vi "SetTreeTags__slk_mt.vi"(8 "error in (no error)":errorcluster, 9 "parents symbol (-)":string="-", 10 "tags in":string[](array[string]), 11 "tree view in":refnum<class "TreeView__slk_mt.lvclass">) -> (0 "error out":errorcluster, 3 "tree view out":refnum<class "TreeView__slk_mt.lvclass">)   [LabVIEW 2020, in "TreeView__slk_mt.lvclass"]
doc: "Sets tags to a tree view objects."
uses:
  TreeView__slk_mt.lvclass
  TreeView__slk_mt.lvclass/TreeView__slk_mt.ctl
panel:
  # "SetTreeTags__slk_mt.vi\nSets tags to a tree view objects.\n\nNOTICE -- YOU MUST LEAVE THIS NOTICE IN PLACE.\n\nCopyright (c) 2011, LIANG LIU Shawn.Liu.cn@gmail.com\nAll rights reserved.\n\nRedistribution and use in source and binary forms, with or without modification, are permitted provided that the following conditions are met:\n-Redistributions of source code must retain the above copyright notice, this list of conditions and the following disclaimer.\n-Redistributions in binary form must reproduce the above copyright notice, this list of conditions and the following disclaimer in the documentation and/or other materials provided with the distribution.\n-Neither the name of the eLp nor the names of its contributors may be used to endorse or promote products derived from this software without specific prior written permission.\n\nTHIS SOFTWARE IS PROVIDED BY THE COPYRIGHT HOLDERS AND CONTRIBUTORS \"AS IS\" AND ANY EXPRESS OR IMPLIED WARRANTIES, INCLUDING, BUT NOT LIMITED TO, THE IMPLIED WARRANTIES OF MERCHANTABILITY AND FITNESS FOR A PARTICULAR PURPOSE ARE DISCLAIMED. IN NO EVENT SHALL THE COPYRIGHT HOLDER OR CONTRIBUTORS BE LIABLE FOR ANY DIRECT, INDIRECT, INCIDENTAL, SPECIAL, EXEMPLARY, OR CONSEQUENTIAL DAMAGES (INCLUDING, BUT NOT LIMITED TO, PROCUREMENT OF SUBSTITUTE GOODS OR SERVICES; LOSS OF USE, DATA, OR PROFITS; OR BUSINESS INTERRUPTION) HOWEVER CAUSED AND ON ANY THEORY OF LIABILITY, WHETHER IN CONTRACT, STRICT LIABILITY, OR TORT (INCLUDING NEGLIGENCE OR OTHERWISE) ARISING IN ANY WAY OUT OF THE USE OF THIS SOFTWARE, EVEN IF ADVISED OF THE POSSIBILITY OF SUCH DAMAGE."
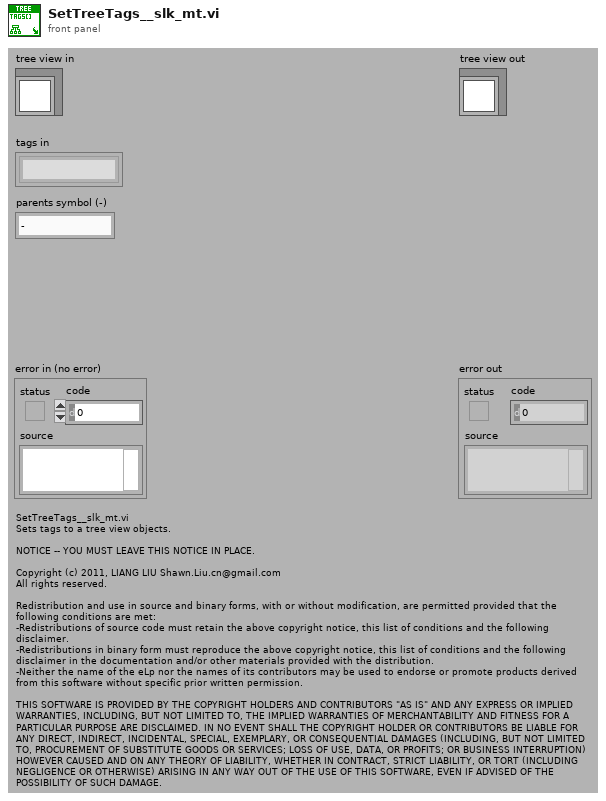
[diagram p1: front panel]
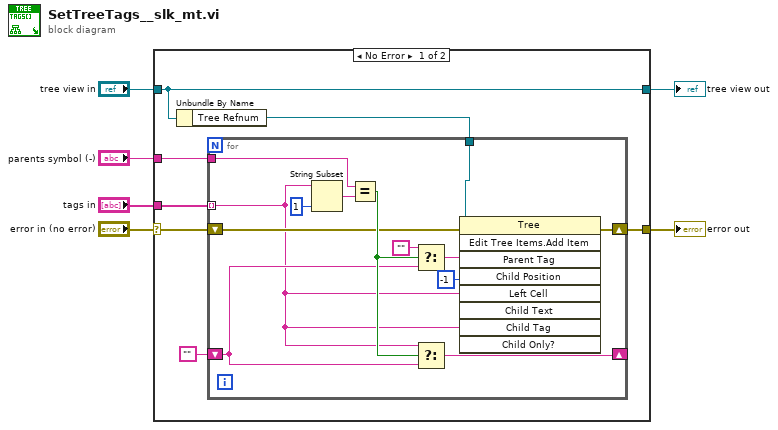
[diagram p0: block diagram]
diagram:
  n1 = case shown="No Error" "error in (no error)" {
    selector: "error in (no error)" -> [w9 w28]
    tunnel: [w11 w28] -> w5
    tunnel: [w13 w27] -> w3
    tunnel: "tree view in" -> [w13 w27]
    tunnel: "tags in" -> [w8 _]
    tunnel: "parents symbol (-)" -> [w7 _]
    frame No Error {
      n2 = Unbundle By Name(w13) -> ("Tree Refnum"=w10:refnum<vi>)
      n3 = for {
        tunnel: w8 -> [w15] mode=indexing
        shift-right: [w24] -> w11
        shift-left: w9 -> [w16]
        shift-right: [w21] -> _
        shift-left: "" -> [w19]
        tunnel: w10 -> [w18]
        tunnel: w7 -> [w14]
        n4 = String Subset(string=w15, length (rest)=1 ("length (rest)")) -> (substring=w25:string)  [unwired: 1 in]
        n5 = Equal?(x=w14, y=w25) -> (x = y?=w20:bool)
        n6 = Select(t="", s=w20, f=w19) -> (s? t:f=w22:string)
        n7 = Select(t=w15, s=w20, f=w19) -> (s? t:f=w21:string)
        n8 = invoke class="Tree" method="Edit Tree Items.Add Item"(reference=w18, error in=w16, "Parent Tag"=w22, "Child Position"=-1, "Left Cell"=w15, "Child Tag"=w15) -> (error out=w24:errorcluster)  [unwired: 3 in, 8 out]
      }
    }
    frame Error {
    }
  }
  "error out" <- w5
  "tree view out" <- w3
